vi "Store Last Deployed.vi"(8 "error in (no error)":errorcluster, 9 "PicoG-Core:DeployResource":refnum<class "DeployResource.lvclass">, 10 "PicoG-Core:DeployTarget":refnum<class "DeployPlatform.lvclass">, 11 "TargetPluginManager in":refnum<class "PlatformPluginManager.lvclass">) -> (0 "error out":errorcluster, 3 "TargetPluginManager out":refnum<class "PlatformPluginManager.lvclass">)   [LabVIEW 2020, in "PicoG-Core.lvlib" / "PlatformPluginManager.lvclass"]
uses:
  PlatformPluginManager.lvclass
  DeployPlatform/DeployPlatform.lvclass
  DeployResource/DeployResource.lvclass
  PlatformPluginManager.lvclass/PlatformPluginManager.ctl
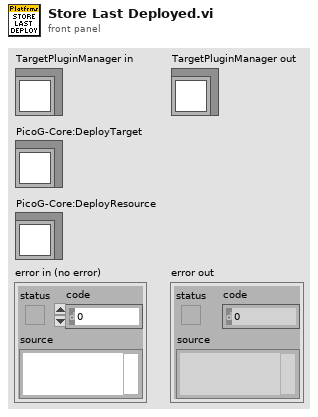
[diagram p1: front panel]
types:
  T1 = typedef "PicoG-Core.lvlib/PlatformPluginManager.lvclass/Ref Data.ctl" = cluster{"Platforms":refnum<class "DeployPlatform.lvclass">[], "Last Platform":refnum<class "DeployPlatform.lvclass">, "Last Resource":refnum<class "DeployResource.lvclass">}
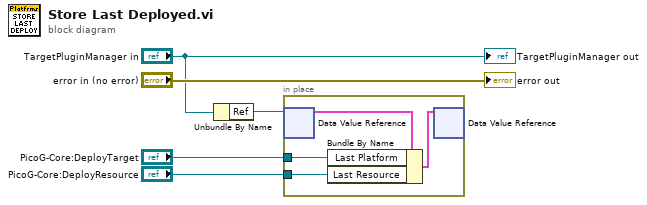
[diagram p0: block diagram]
diagram:
  n1 = Unbundle By Name("TargetPluginManager in") -> ("Ref"=w4:refnum<data-value>)
  n2 = in-place {
    in-place-border: "PicoG-Core:DeployTarget" -> [w7]
    in-place-border: "PicoG-Core:DeployResource" -> [w6]
    n3 = in-place-dvr #1(w4) -> (w9:T1)  [unwired: 1 out]
    n4 = Bundle By Name(cluster=w9, "Last Platform"=w7, "Last Resource"=w6) -> (w8:T1)
    n5 = in-place-dvr #1(w8) -> ()  [unwired: 2 out]
  }
  "error out" <- "error in (no error)"
  "TargetPluginManager out" <- "TargetPluginManager in"
